vi "Get Service Class Instances.vi"() -> (3 "service instances":refnum<class "ServiceBase.lvclass">[](array[class]))   [LabVIEW 2025, in "reflection_server.lvlib"]
uses:
  reflection_server.lvlib
  <vilib>/gRPC/LabVIEW gRPC Servicer/ServiceBase/ServiceBase.lvclass
  RPC Service/ServerReflection/ServerReflection.lvclass
  C:/Program Files/National Instruments/LabVIEW 2025/vi.lib/gRPC/LabVIEW gRPC Servicer/ServiceBase/ServiceBase.lvclass
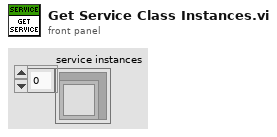
[diagram p1: front panel]
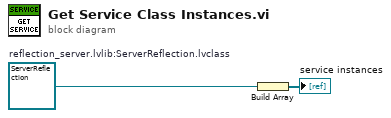
[diagram p0: block diagram]
diagram:
  w1 = refnum<class "ServerReflection.lvclass"> refnum  # reflection_server.lvlib:ServerReflection.lvclass
  n1 = Build Array(w1) -> (→"service instances":refnum<class "ServerReflection.lvclass">[])
